vi "Get Categories.vi"(8 "error in (no error)":errorcluster, 11 "Budgetizer in":refnum<class "Budgetizer.lvclass">) -> (0 "error out":errorcluster, 2 "All Categories":refnum<class "Category.lvclass">[](array[class]), 3 "Budgetizer out":refnum<class "Budgetizer.lvclass">)   [LabVIEW 2018, in "Budgetizer.lvclass"]
uses:
  Budgetizer.lvclass
  Category/Category.lvclass
  Budgetizer.lvclass/Budgetizer.ctl
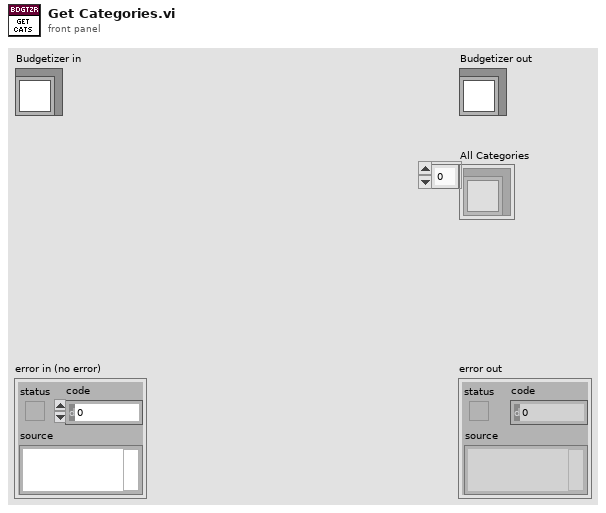
[diagram p1: front panel]
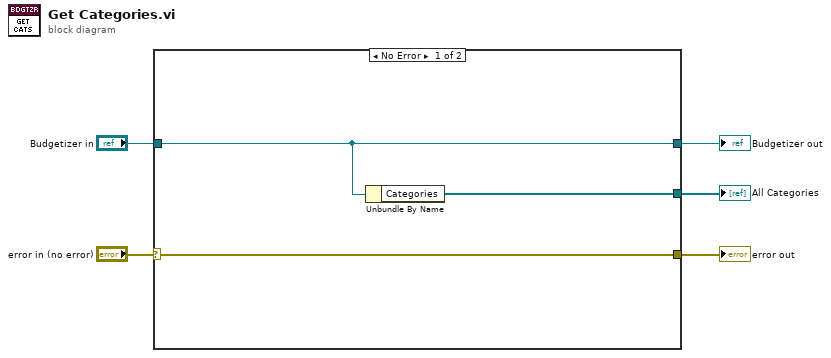
[diagram p0: block diagram]
diagram:
  n1 = case shown="No Error" "error in (no error)" {
    selector: "error in (no error)" -> [w6 w10]
    tunnel: [w6 w10] -> w4
    tunnel: [w8 w9] -> w2
    tunnel: "Budgetizer in" -> [w8 w9]
    tunnel: [w7 _] -> w1
    frame No Error {
      n2 = Unbundle By Name(w8) -> ("Categories"=w7:refnum<class "Category.lvclass">[])
    }
    frame Error {
    }
  }
  "error out" <- w4
  "Budgetizer out" <- w2
  "All Categories" <- w1
